vi "Example.vi"() -> ()   [LabVIEW 2016, in "Timer Session.lvclass"]
uses:
  Timer Session.lvclass
panel:
  out "Time Goal (s)":dbl format="%#.6f"
  out "Elapsed Time 3":dbl format="%#_4p"
  out "Elapsed Time 2":dbl format="%#_4p"
  out "Elapsed Time 1":dbl format="%_4p"
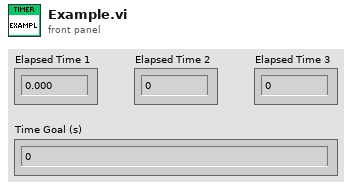
[diagram p1: front panel]
types:
  T1 = typedef "Timer Session.lvclass/Session Handle.ctl" = refnum<data-value>
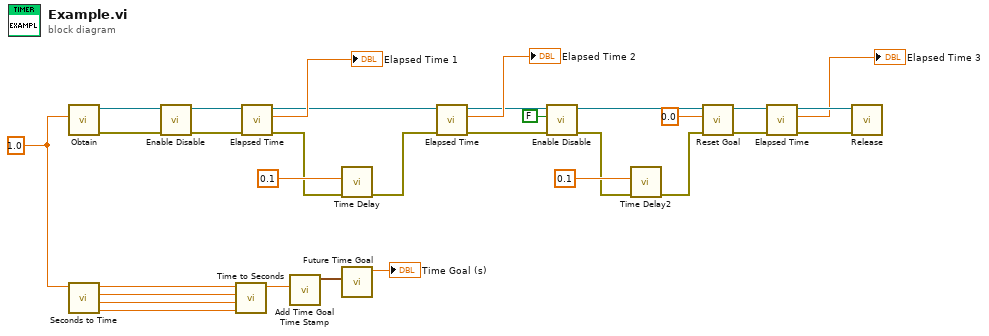
[diagram p0: block diagram]
diagram:
  w29 = 1.0 ("Time Goal (s)")
  n1 = call "Obtain.vi"("Time Goal (s)"=w29) -> ("Error Out"=w1:errorcluster, "Timer Handle"=w4:T1)  [unwired: 9 in]
  n2 = call "Seconds to Time.vi"("Time Goal (s)"=w29) -> ("Seconds"=w25:dbl, "Minutes"=w26:dbl, "Hours"=w27:dbl, "Days"=w28:dbl)  [unwired: 7 in]
  n3 = call "Enable Disable.vi"("Error In"=w1, "Timer Handle"=w4) -> ("Error Out"=w2:errorcluster, "Timer Handle"=w3:T1)  [unwired: 8 in]
  n4 = call "Time to Seconds.vi"("Seconds"=w25, "Minutes"=w26, "Hours"=w27, "Days"=w28) -> ("Time Goal (s)"=w24:dbl)  [unwired: 7 in]
  n5 = call "Elapsed Time.vi"("Error In"=w2, "Timer Handle"=w3) -> ("Error Out"=w15:errorcluster, "Elapsed Time"=→"Elapsed Time 1":dbl, "Timer Handle"=w12:T1)  [unwired: 6 in, 1 out]
  n6 = call "Add Time Goal Time Stamp.vi"("Time Goal (s)"=w24) -> ("Resulting Time"=w23:timestamp)  [unwired: 10 in]
  n7 = call "Time Delay"("error in (no error)"=w15, "Delay Time (s)"=0.1) -> ("error out"=w13:errorcluster)  [unwired: 9 in]
  n8 = call "Future Time Goal.vi"("Future Time"=w23) -> ("Time Goal (s)"=→"Time Goal (s)":dbl)  [unwired: 10 in]
  n9 = call "Elapsed Time.vi"("Error In"=w13, "Timer Handle"=w12) -> ("Error Out"=w11:errorcluster, "Elapsed Time"=→"Elapsed Time 2":dbl, "Timer Handle"=w9:T1)  [unwired: 6 in, 1 out]
  n10 = call "Enable Disable.vi"("Error In"=w11, "Enable (T)"=FALSE, "Timer Handle"=w9) -> ("Error Out"=w7:errorcluster, "Timer Handle"=w8:T1)  [unwired: 7 in]
  n11 = call "Time Delay2"("error in (no error)"=w7, "Delay Time (s)"=0.1) -> ("error out"=w6:errorcluster)  [unwired: 9 in]
  n12 = call "Reset Goal.vi"("Error In"=w6, "Time Goal (s)"=0.0, "Timer Handle"=w8) -> ("Error Out"=w19:errorcluster, "Timer Handle"=w20:T1)  [unwired: 7 in]
  n13 = call "Elapsed Time.vi"("Error In"=w19, "Timer Handle"=w20) -> ("Error Out"=w18:errorcluster, "Elapsed Time"=→"Elapsed Time 3":dbl, "Timer Handle"=w17:T1)  [unwired: 6 in, 1 out]
  n14 = call "Release.vi"("Error In"=w18, "Timer Handle"=w17) -> ()  [unwired: 8 in, 2 out]
